vi "Periodic Tasks.vi"(8 "error in":errorcluster) -> ()   [LabVIEW 2018]
doc: "This VI runs in parallel to other robot code. It can contain as many user-defined periodic loops as you need. These can carry out PID or other sorts of timed response."
uses:
  Robot Global Data.vi
panel:
  out "Average Voltage":dbl
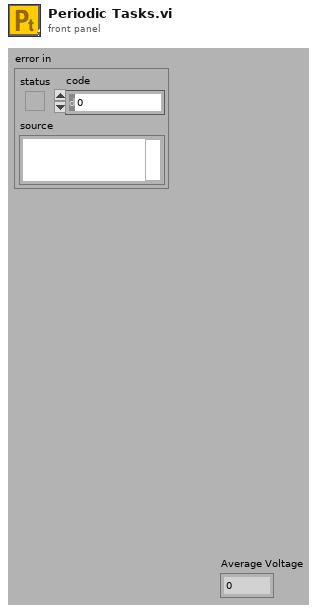
[diagram p1: front panel]
types:
  T1 = typedef "WPI_JoystickDevRef.ctl" = cluster{"Device":T2}
  T2 = typedef "WPI_JoystickDeviceEnum.ctl" = enum16{"USB 0", "USB 1", "USB 2", "USB 3", "USB 4", "USB 5"}
  T3 = typedef "WPI_AnalogChannelDevRef.ctl" = cluster{"DevStatus":errorcluster, "Analog Channel":T4}
  T4 = typedef "FPGA_AIChannel.ctl" = enum8{"AI 0", "AI 1", "AI 2", "AI 3", "AI MXP 0", "AI MXP 1", "AI MXP 2", "AI MXP 3", "Invalid"}
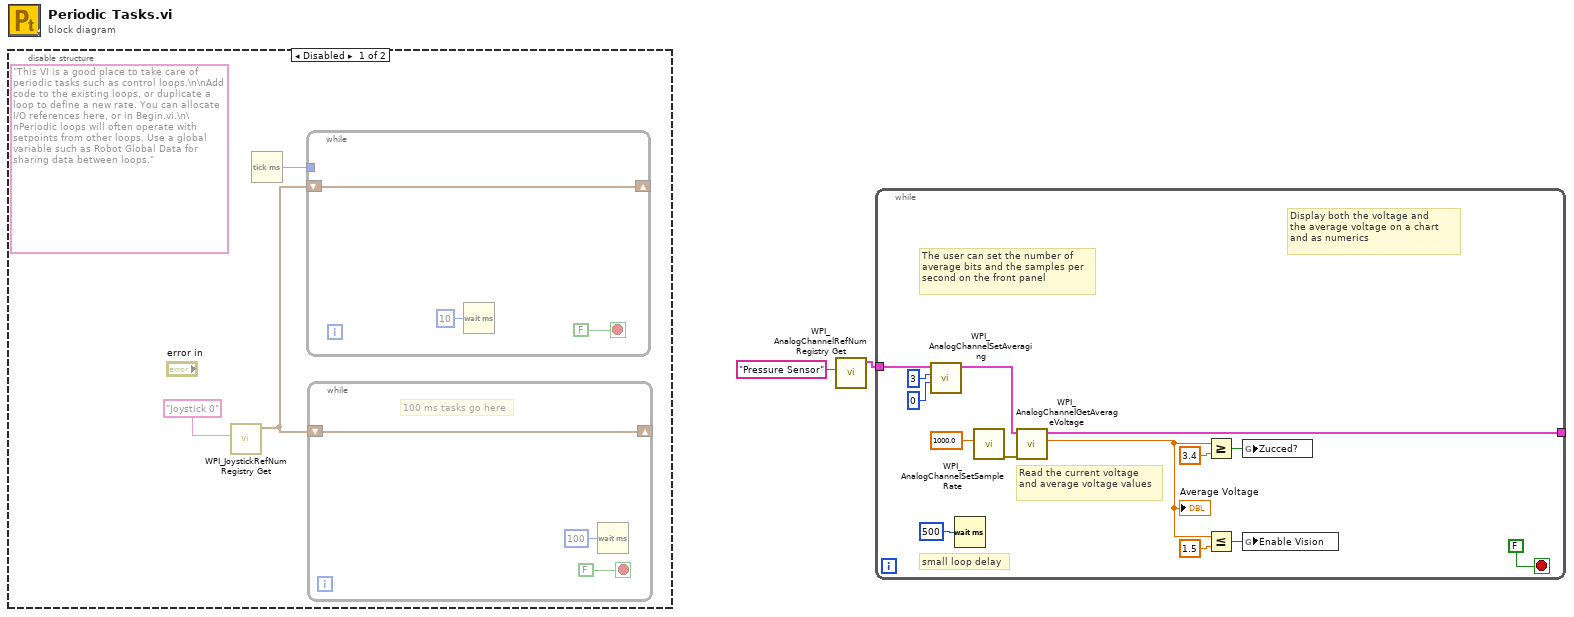
[diagram p0: block diagram]
diagram:
  n1 = disable-structure shown="Disabled" {
    frame Disabled {
      (unwired) "This VI is a good place to take care of periodic tasks such as control loops.\n\nAdd code to the existing loops, or duplicate a loop to define a new rate. You can allocate I/O references here, or in Begin.vi.\n\nPeriodic loops will often operate with setpoints from other loops. Use a global variable such as Robot Global Data for sharing data between loops."
      n2 = call <vilib>:"WPI_JoystickRefNum Registry Get.vi"("refnum name"="Joystick 0") -> ("JoystickDevRef"=w4:T1)  [unwired: 1 in, 9 out]
      n3 = Tick Count (ms)() -> (millisecond timer value=w3:u32)
      n4 = while {
        shift-right: [w10] -> _
        shift-left: w4 -> [w10]
        tunnel: w3 -> [_]
        stop <- FALSE stop-if-true
        n5 = Wait (ms)(milliseconds to wait=u32 10) -> ()  [unwired: 1 out]
      }
      n6 = while {
        shift-right: [w6] -> _
        shift-left: w4 -> [w6]
        stop <- FALSE stop-if-true
        # "100 ms tasks go here"
        n7 = Wait (ms)(milliseconds to wait=u32 100) -> ()  [unwired: 1 out]
      }
    }
    frame Enabled {
    }
  }
  n8 = call <vilib>:"WPI_AnalogChannelRefNum Registry Get.vi"("refnum name"="Pressure Sensor") -> ("AIDeviceRef"=w2:T3)  [unwired: 9 in, 1 out]
  n9 = while {
    tunnel: w2 -> [w23]
    tunnel: [w25] -> _
    stop <- FALSE stop-if-true
    # "small loop delay"
    # "Read the current voltage\nand average voltage values"
    # "Display both the voltage and\nthe average voltage on a chart\nand as numerics"
    # "The user can set the number of \naverage bits and the samples per\nsecond on the front panel"
    n10 = call <vilib>:"WPI_AnalogChannelSetAveraging.vi"("OversampleBits"=u8 0, "AverageBits"=u8 3 ("Average Bits"), "AIDeviceRef"=w23) -> ("AIDeviceRef"=w19:T3)  [unwired: 1 in, 7 out]
    n11 = Wait (ms)(milliseconds to wait=u32 500) -> ()  [unwired: 1 out]
    n12 = call <vilib>:"WPI_AnalogChannelSetSampleRate.vi"("Samples Per Second (per channel)"=1000.0 ("Samples Per Second")) -> ("error out"=w17:errorcluster)  [unwired: 4 in, 6 out]
    n13 = call <vilib>:"WPI_AnalogChannelGetAverageVoltage.vi"("error in (no error)"=w17, "AIDeviceRef"=w19) -> ("Voltage"=w13:dbl, "AIDeviceRef"=w25:T3)  [unwired: 8 out]
    "Average Voltage" <- w13
    n14 = Greater Or Equal?(x=w13, y=3.4) -> (x >= y?=w15:bool)
    n15 = Less Or Equal?(x=w13, y=1.5) -> (x <= y?=w12:bool)
    n16 = global write "Robot Global Data.vi" "Zucced?"(w15) -> ()
    n17 = global write "Robot Global Data.vi" "Enable Vision"(w12) -> ()
  }
